vi "Periodic Tasks.vi"(8 "error in":errorcluster) -> ()   [LabVIEW 2013]
doc: "This VI runs in parallel to other tasks. It can contain as many user-defined periodic loops as you need. These can carry out PID or other sorts of timed response."
uses:
  <vilib>/Rock Robotics/WPI/DriverStation/DriverStationLCD/WPI_DriverStationLCDLCDLine.ctl
  <vilib>/Rock Robotics/SystemInterfaces/Utilities/FPGA_UtilitiesLED Source.ctl
  <vilib>/Rock Robotics/SystemInterfaces/Utilities/FPGA_UtilitiesLED State.ctl
  <vilib>/Rock Robotics/WPI/Relay/WPI_RelayValue.ctl
  <vilib>/Rock Robotics/WPI/SafetyOutput/WPI_SafetyOutputConfigMenu.ctl
  <vilib>/Rock Robotics/WPI/DriverStation/WPI_DriverStationRobotMode2.ctl
  <vilib>/Rock Robotics/WPI/Solenoid/WPI_SolenoidValue.ctl
  Begin/Global Refnums.vi
  <vilib>/Rock Robotics/WPI/Solenoid/WPI_SolenoidSetEnum.vi
  Begin/Robot Global Data.vi
  Begin/Global Variables.vi
  <vilib>/Rock Robotics/WPI/Joystick/WPI_JoystickGetSetRefNum.vi
  <vilib>/Rock Robotics/WPI/Compressor/WPI_CompressorGetSetRefNum.vi
panel:
  out "Fire":bool
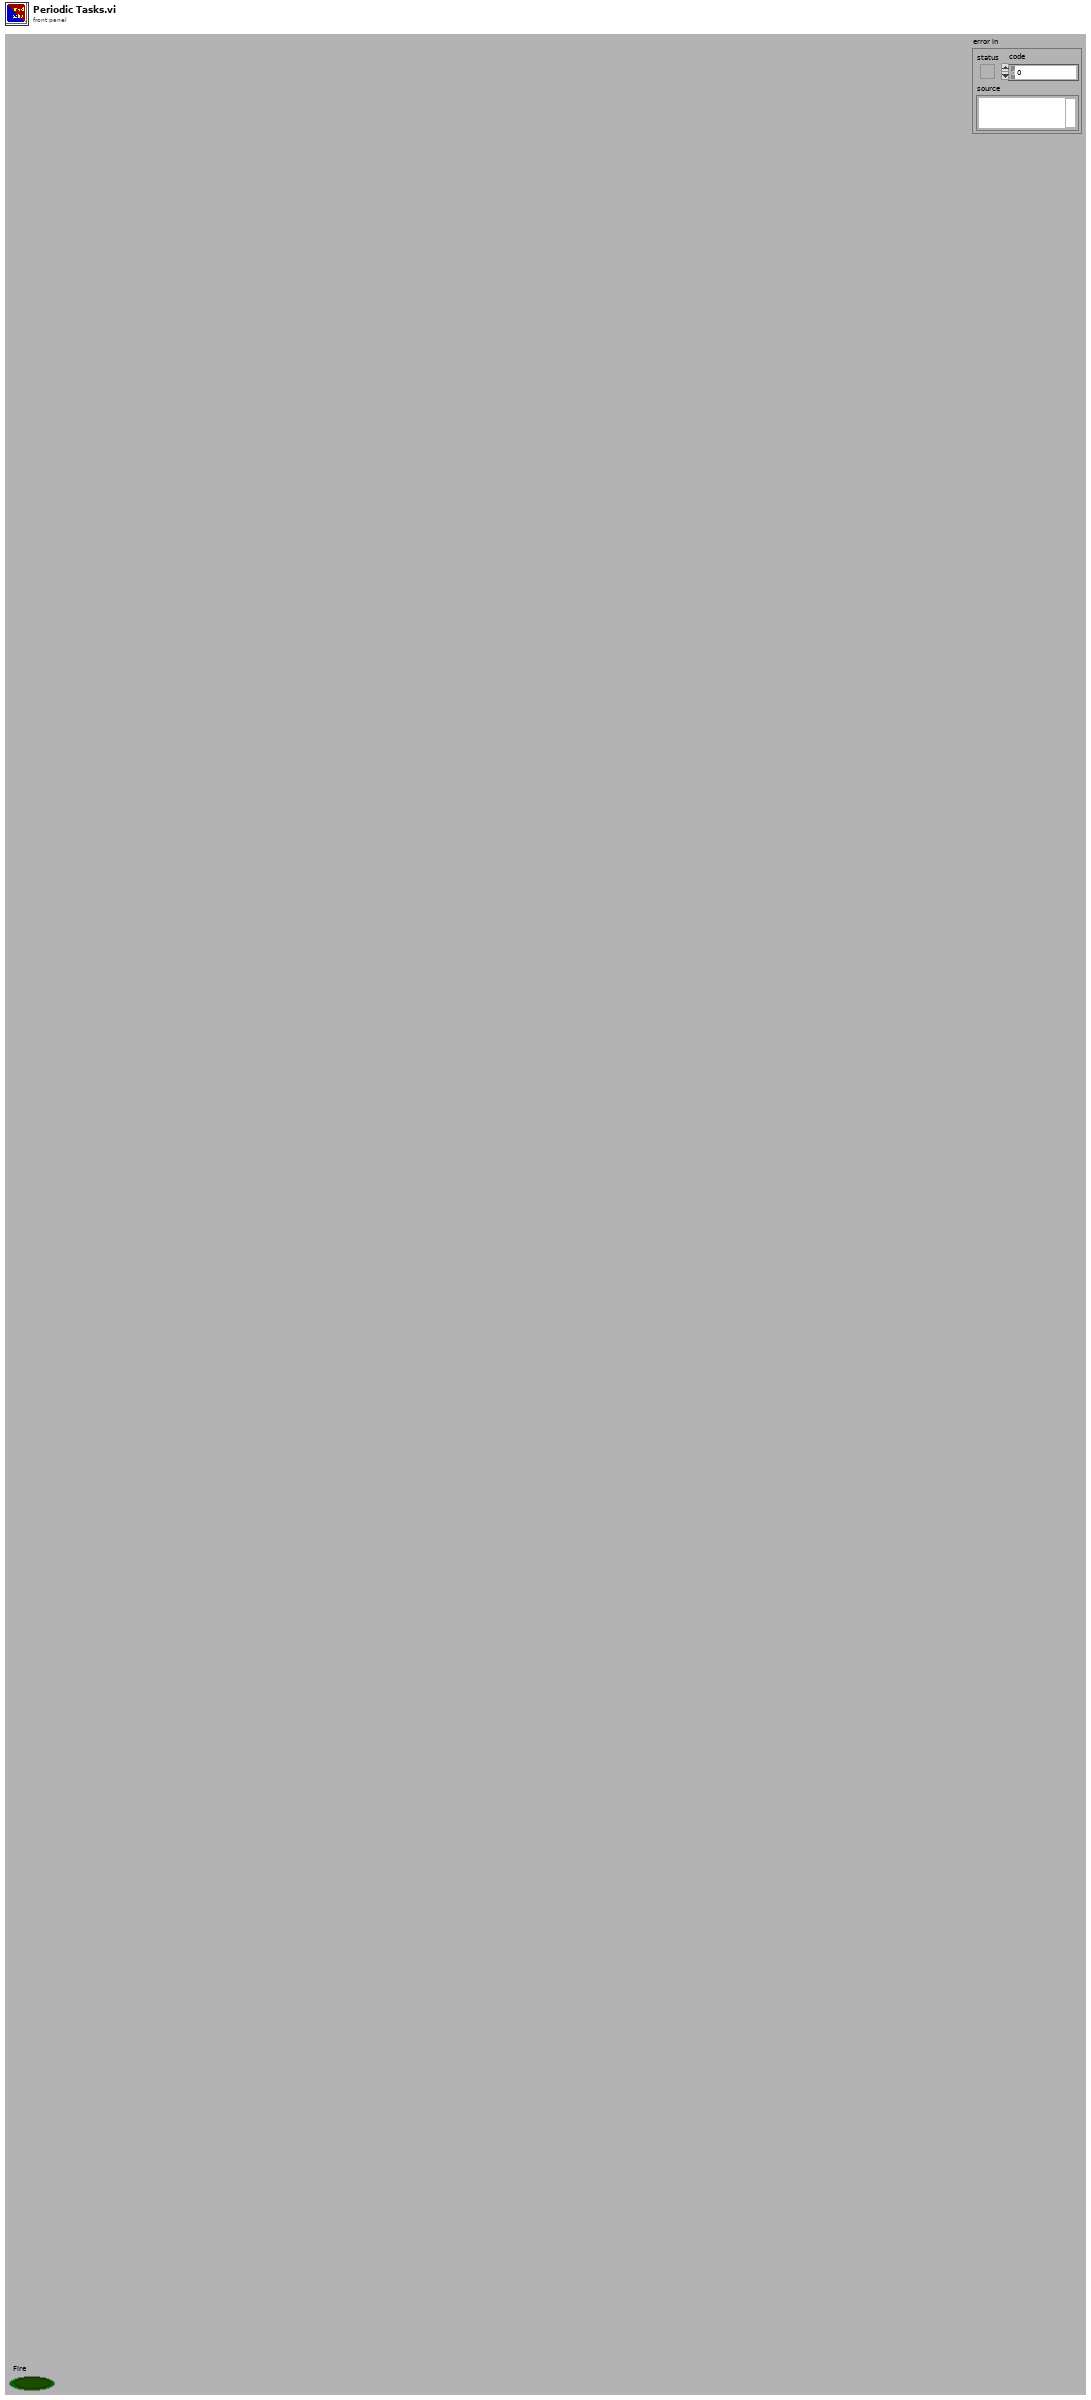
[diagram p1: front panel]
types:
  T1 = typedef "WPI_DriverStationLCDLCDLine.ctl" = enum16{"Main - Line 1", "User - Line 2", "User - Line 3", "User - Line 4", "User - Line 5", "User - Line 6"}
  T2 = typedef "WPI_CompressorDevRef.ctl" = cluster{"DevStatus":errorcluster, "DigitalInputDevRef":T3, "RelayDevRef":T6}
  T3 = typedef "WPI_DigitalInputDevRef.ctl" = cluster{"DevStatus":errorcluster, "DIO Channel":T4, "Digital Module":T5}
  T4 = typedef "FPGA_DIOChannel.ctl" = enum8{"DIO 1", "DIO 2", "DIO 3", "DIO 4", "DIO 5", "DIO 6", "DIO 7", "DIO 8", "DIO 9", "DIO 10", "DIO 11", "DIO 12", "DIO 13", "DIO 14", "Invalid"}
  T5 = typedef "FPGA_TypedefDigitalModule.ctl" = enum16{"Digital Module 1", "Digital Module 2"}
  T6 = typedef "WPI_RelayDevRef.ctl" = cluster{"DevStatus":errorcluster, "Relay Channel":T7, "Digital Module":T5, "Relay Direction":T8}
  T7 = typedef "FPGA_DIORelayChannel.ctl" = enum8{"Relay 1", "Relay 2", "Relay 3", "Relay 4", "Relay 5", "Relay 6", "Relay 7", "Relay 8", "Invalid"}
  T8 = typedef "WPI_RelayDirection.ctl" = enum16{"Both directions", "Forward only", "Reverse only"}
  T9 = typedef "WPI_SolenoidValue.ctl" = enum16{"Off", "On", "Forward", "Reverse"}
  T10 = typedef "WPI_SafetyOutputConfigMenu.ctl" = enum16{"Enable", "Disable"}
  T11 = typedef "WPI_SolenoidDevRef.ctl" = cluster{"DevStatus":errorcluster, "Solenoid Module":T12, "Forward Solenoid Channel":T13, "Reverse Solenoid Channel":T13}
  T12 = typedef "FPGA_TypedefSolenoidModule.ctl" = enum16{"Solenoid Module 1", "Solenoid Module 2"}
  T13 = typedef "WPI_SolenoidChannel.ctl" = enum8{"Solenoid 1", "Solenoid 2", "Solenoid 3", "Solenoid 4", "Solenoid 5", "Solenoid 6", "Solenoid 7", "Solenoid 8", "Invalid"}
  T14 = typedef "WPI_RelayValue.ctl" = enum16{"Off", "On", "Forward", "Reverse"}
  T15 = typedef "WPI_EncoderDevRef.ctl" = cluster{"DevStatus":errorcluster, "EncoderIndex":T16, "CounterIndex":T17, "DistancePerCount":dbl, "Decoding Type":T18}
  T16 = typedef "FPGA_EncoderIdx.ctl" = enum8{"Enc 0", "Enc 1", "Enc 2", "Enc 3", "Invalid"}
  T17 = typedef "FPGA_CounterCtrSystemIndex.ctl" = enum8{"Ctr 0", "Ctr 1", "Ctr 2", "Ctr 3", "Ctr 4", "Ctr 5", "Ctr 6", "Ctr 7", "Invalid"}
  T18 = typedef "WPI_EncoderType.ctl" = enum16{"1x", "2x", "4x"}
  T19 = typedef "WPI_DriverStationRobotMode2.ctl" = enum16{"Autonomous Disabled", "Autonomous Enabled", "Teleop Disabled", "Teleop Enabled", "Timeout", "Finish", "Test Disabled", "Test Enabled"}
  T20 = typedef "WPI_JoystickDevRef.ctl" = cluster{"Device":T21}
  T21 = typedef "WPI_JoystickDeviceEnum.ctl" = enum16{"USB 1", "USB 2", "USB 3", "USB 4", "Kinect 1", "Kinect 2"}
  T22 = typedef "WPI_JoystickButtonState.ctl" = cluster{"Button 1":bool, "Button 2":bool, "Button 3":bool, "Button 4":bool, "Button 5":bool, "Button 6":bool, "Button 7":bool, "Button 8":bool, "Button 9":bool, "Button 10":bool, "Button 11":bool, "Button 12":bool}
  T23 = typedef "WPI_MotorControlDeviceRef.ctl" = cluster{"DeviceStatus":errorcluster, "Type":enum16{"PWM", "CAN"}, "PWM":cluster{"Digital Module":T5, "PWM Channel":T24, "DeadBand":T25}, "CAN":cluster{"Device Number":u8, "Control Mode":T26, "Semaphore":T27, "Max Vout":dbl}, "Invert":bool, "TransformRef":T28, "InvTransformRef":T28}
  T24 = typedef "FPGA_DIOPWMChannel.ctl" = enum8{"PWM 1", "PWM 2", "PWM 3", "PWM 4", "PWM 5", "PWM 6", "PWM 7", "PWM 8", "PWM 9", "PWM 10", "Invalid"}
  T25 = typedef "WPI_PWMDeadband.ctl" = cluster{"Name":string, "maxPositivePwm":i32, "minPositivePwm":i32, "centerPwm":i32, "maxNegativePwm":i32, "minNegativePwm":i32, "angularRange":u16}
  T26 = typedef "WPI_CANJaguar_ControlMode.ctl" = enum8{"Percent VBus", "Current", "Speed", "Position", "Voltage"}
  T27 = typedef "Semaphore RefNum" = refnum<k1>
  T28 = typedef "WPI_PWMTransform_ConPane.ctl" = refnum<vi>
  T29 = typedef "FPGA_UtilitiesLED State.ctl" = enum16{"Off", "On", "Toggle"}
  T30 = typedef "FPGA_UtilitiesLED Source.ctl" = enum16{"User LED", "FPGA LED"}
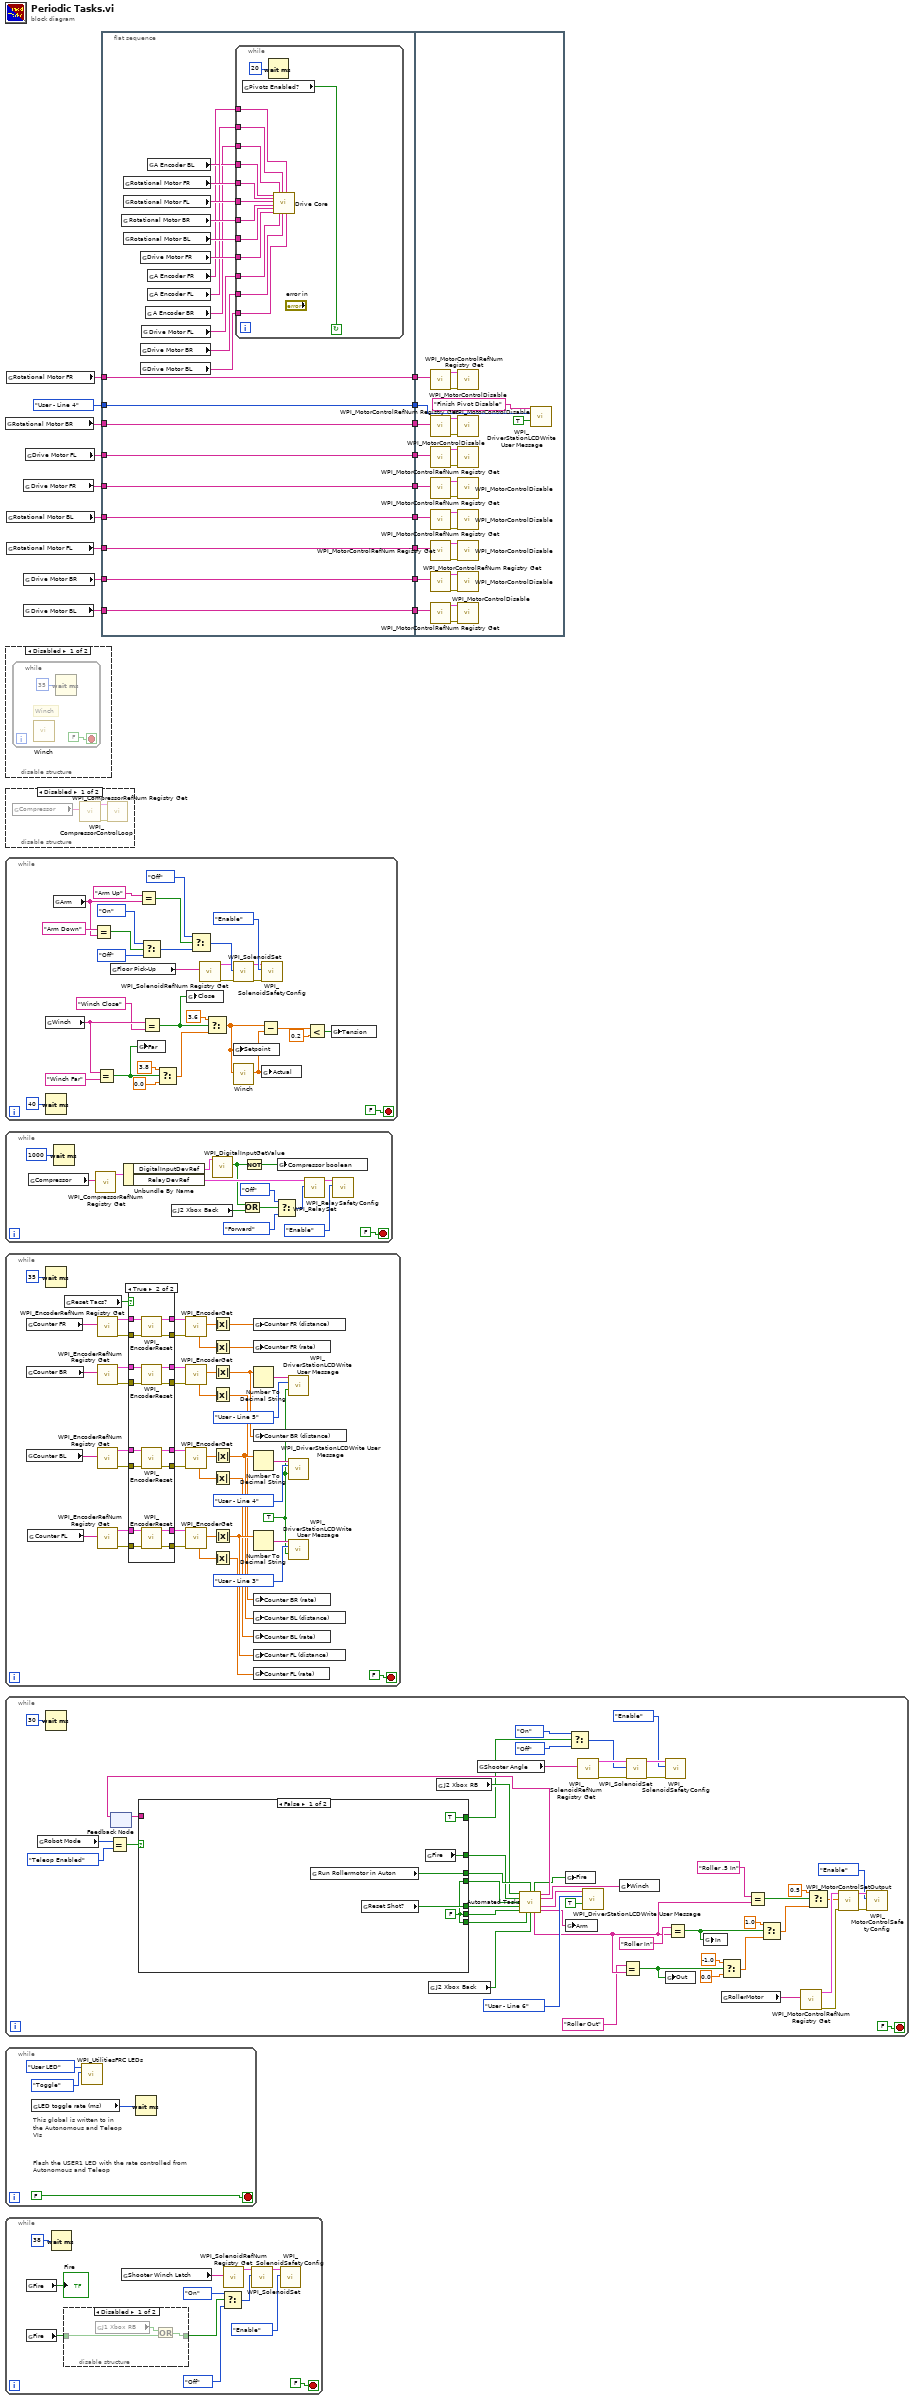
[diagram p0: block diagram]
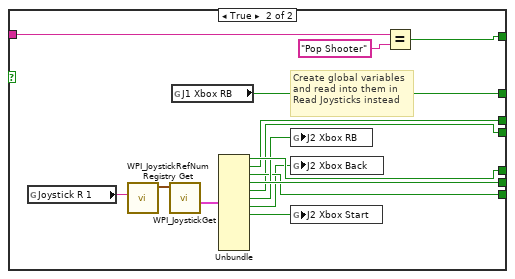
[diagram p4: hidden frame]
diagram:
  n1 = global read "Global Refnums.vi" "Rotational Motor BR"() -> (w16:string)
  n2 = disable-structure shown="Disabled" {
    frame Disabled {
      n3 = while {
        stop <- FALSE stop-if-true
        # "Winch"
        n4 = call "Winch.vi"() -> ()  [unwired: 11 in, 1 out]
        n5 = Wait (ms)(milliseconds to wait=u32 35) -> ()  [unwired: 1 out]
      }
    }
    frame Enabled {
    }
  }
  n6 = disable-structure shown="Disabled" {
    frame Disabled {
      n7 = global read "Global Refnums.vi" "Compressor"() -> (w23:string)
      n8 = call <vilib>:"WPI_CompressorRefNum Registry Get.vi"("refnum name"=w23) -> ("error out"=w22:errorcluster, "CompressorDevRef"=w21:T2)  [unwired: 9 in]
      n9 = call <vilib>:"WPI_CompressorControlLoop.vi"("error in (no error)"=w22, "CompressorDevRef"=w21) -> ()  [unwired: 10 in]
    }
    frame Enabled {
    }
  }
  n10 = while {
    stop <- FALSE stop-if-true
    n11 = global read "Global Refnums.vi" "Winch"() -> (w55:string)
    n12 = Wait (ms)(milliseconds to wait=u32 40) -> ()  [unwired: 1 out]
    n13 = global read "Global Refnums.vi" "Arm"() -> (w29:string)
    n14 = Equal?(x="Arm Down", y=w29) -> (x = y?=w33:bool)
    n15 = Equal?(x=w55, y="Winch Far") -> (x = y?=w26:bool)
    n16 = global read "Global Refnums.vi" "Floor Pick-Up"() -> (w44:string)
    n17 = global write "Global Refnums.vi" "Far"(w26) -> ()
    n18 = Equal?(x="Arm Up", y=w29) -> (x = y?=w46:bool)
    n19 = Select(t=WPI_SolenoidValue."On" ("Value"), s=w33, f=WPI_SolenoidValue."Off" ("Value")) -> (s? t:f=w32:T9)
    n20 = Equal?(x=w55, y="Winch Close") -> (x = y?=w25:bool)
    n21 = Select(t=3.8, s=w26, f=0.0) -> (s? t:f=w52:dbl)
    n22 = global write "Global Refnums.vi" "Close"(w25) -> ()
    n23 = Select(t=WPI_SolenoidValue."Off" ("Value"), s=w46, f=w32) -> (s? t:f=w48:T9)
    n24 = call <vilib>:"WPI_SolenoidRefNum Registry Get.vi"("refnum name"=w44) -> ("error out"=w39:errorcluster, "SolenoidDevRef"=w40:T11)  [unwired: 9 in]
    n25 = Select(t=3.6, s=w25, f=w52) -> (s? t:f=w24:dbl)
    n26 = call-poly <vilib>:"WPI_SolenoidSet.vi"("error in (no error)"=w39, "Value"=w48, "SolenoidDevRef"=w40) -> ("error out"=w42:errorcluster, "SolenoidDevRef"=w41:T11)  [unwired: 7 in]
    n27 = global write "Global Refnums.vi" "Setpoint"(w24) -> ()
    n28 = call "Winch.vi"("setpoint"=w24) -> ("Actual"=w27:dbl)  [unwired: 10 in]
    n29 = Subtract(x=w24, y=w27) -> (x-y=w36:dbl)
    n30 = call <vilib>:"WPI_SolenoidSafetyConfig.vi"("error in (no error)"=w42, "mode"=WPI_SafetyOutputConfigMenu."Enable", "SolenoidDevRef"=w41) -> ()  [unwired: 7 in, 2 out]
    n31 = global write "Global Refnums.vi" "Actual"(w27) -> ()
    n32 = Less?(x=w36, y=0.2) -> (x < y?=w28:bool)
    n33 = global write "Global Refnums.vi" "Tension"(w28) -> ()
  }
  n34 = while {
    stop <- FALSE stop-if-true
    n35 = global read "Global Refnums.vi" "Compressor"() -> (w68:string)
    n36 = Wait (ms)(milliseconds to wait=1000) -> ()  [unwired: 1 out]
    n37 = call <vilib>:"WPI_CompressorRefNum Registry Get.vi"("refnum name"=w68) -> ("CompressorDevRef"=w67:T2)  [unwired: 9 in, 1 out]
    n38 = Unbundle By Name(w67) -> ("DigitalInputDevRef"=w60:T3, "RelayDevRef"=w66:T6)
    n39 = global read "Global Variables.vi" "J2 Xbox Back"() -> (w58:bool)
    n40 = call <vilib>:"WPI_DigitalInputGetValue.vi"("DigitalInputDevRef"=w60) -> ("Value"=w57:bool)  [unwired: 8 in, 2 out]
    n41 = Or(x=w57, y=w58) -> (x .or. y?=w59:bool)
    n42 = Not(x=w57) -> (.not. x?=w56:bool)
    n43 = Select(t=WPI_RelayValue."Off" ("RelayValue"), s=w59, f=WPI_RelayValue."Forward" ("RelayValue")) -> (s? t:f=w63:T14)
    n44 = global write "Global Refnums.vi" "Compressor boolean"(w56) -> ()
    n45 = call <vilib>:"WPI_RelaySet.vi"("RelayValue"=w63, "RelayDevRef"=w66) -> ("RelayDevRef"=w65:T6)  [unwired: 8 in, 1 out]
    n46 = call <vilib>:"WPI_RelaySafetyConfig.vi"("mode"=WPI_SafetyOutputConfigMenu."Enable", "RelayDevRef"=w65) -> ()  [unwired: 8 in, 2 out]
  }
  n47 = while {
    stop <- FALSE stop-if-true
    w72 = TRUE ("clear line before write (T)")
    n48 = global read "Global Refnums.vi" "Counter FR"() -> (w83:string)
    n49 = global read "Global Refnums.vi" "Counter BR"() -> (w81:string)
    n50 = global read "Global Refnums.vi" "Counter BL"() -> (w84:string)
    n51 = global read "Global Refnums.vi" "Counter FL"() -> (w82:string)
    n52 = Wait (ms)(milliseconds to wait=u32 35) -> ()  [unwired: 1 out]
    n53 = global read "Global Variables.vi" "Reset Tacs?"() -> (w71:bool)
    n54 = call <vilib>:"WPI_EncoderRefNum Registry Get.vi"("refnum name"=w83) -> ("error out"=w99:errorcluster, "EncoderDevRef"=w102:T15)  [unwired: 9 in]
    n55 = call <vilib>:"WPI_EncoderRefNum Registry Get.vi"("refnum name"=w81) -> ("error out"=w107:errorcluster, "EncoderDevRef"=w108:T15)  [unwired: 9 in]
    n56 = call <vilib>:"WPI_EncoderRefNum Registry Get.vi"("refnum name"=w84) -> ("error out"=w109:errorcluster, "EncoderDevRef"=w110:T15)  [unwired: 9 in]
    n57 = call <vilib>:"WPI_EncoderRefNum Registry Get.vi"("refnum name"=w82) -> ("error out"=w104:errorcluster, "EncoderDevRef"=w105:T15)  [unwired: 9 in]
    n58 = case shown="True" w71 {
      tunnel: w108 -> [w121 w140]
      tunnel: [w121 w139] -> w113
      tunnel: [w123 w138] -> w114
      tunnel: w107 -> [w123 w137]
      tunnel: [w122 w136] -> w112
      tunnel: [w124 w135] -> w111
      tunnel: w110 -> [w122 w134]
      tunnel: w109 -> [w124 w133]
      tunnel: [w120 w125] -> w106
      tunnel: w105 -> [w120 w132]
      tunnel: w104 -> [w119 w131]
      tunnel: [w119 w126] -> w103
      tunnel: w102 -> [w118 w130]
      tunnel: [w118 w127] -> w101
      tunnel: [w117 w128] -> w100
      tunnel: w99 -> [w117 w129]
      frame False {
      }
      frame True {
        n59 = call <vilib>:"WPI_EncoderReset.vi"("error in (no error)"=w129, "EncoderDevRef"=w130) -> ("error out"=w128:errorcluster, "EncoderDevRef"=w127:T15)  [unwired: 8 in]
        n60 = call <vilib>:"WPI_EncoderReset.vi"("error in (no error)"=w137, "EncoderDevRef"=w140) -> ("error out"=w138:errorcluster, "EncoderDevRef"=w139:T15)  [unwired: 8 in]
        n61 = call <vilib>:"WPI_EncoderReset.vi"("error in (no error)"=w133, "EncoderDevRef"=w134) -> ("error out"=w135:errorcluster, "EncoderDevRef"=w136:T15)  [unwired: 8 in]
        n62 = call <vilib>:"WPI_EncoderReset.vi"("error in (no error)"=w131, "EncoderDevRef"=w132) -> ("error out"=w126:errorcluster, "EncoderDevRef"=w125:T15)  [unwired: 8 in]
      }
    }
    n63 = call <vilib>:"WPI_EncoderGet.vi"("error in (no error)"=w100, "EncoderDevRef"=w101) -> ("Distance"=w96:dbl, "Rate"=w92:dbl)  [unwired: 4 in, 4 out]
    n64 = call <vilib>:"WPI_EncoderGet.vi"("error in (no error)"=w114, "EncoderDevRef"=w113) -> ("Distance"=w95:dbl, "Rate"=w91:dbl)  [unwired: 4 in, 4 out]
    n65 = call <vilib>:"WPI_EncoderGet.vi"("error in (no error)"=w111, "EncoderDevRef"=w112) -> ("Distance"=w97:dbl, "Rate"=w93:dbl)  [unwired: 4 in, 4 out]
    n66 = call <vilib>:"WPI_EncoderGet.vi"("error in (no error)"=w103, "EncoderDevRef"=w106) -> ("Distance"=w98:dbl, "Rate"=w94:dbl)  [unwired: 4 in, 4 out]
    n67 = Absolute Value(x=w96) -> (abs(x)=w80:dbl)
    n68 = Absolute Value(x=w92) -> (abs(x)=w79:dbl)
    n69 = Absolute Value(x=w91) -> (abs(x)=w73:dbl)
    n70 = Absolute Value(x=w93) -> (abs(x)=w75:dbl)
    n71 = Absolute Value(x=w94) -> (abs(x)=w77:dbl)
    n72 = Absolute Value(x=w95) -> (abs(x)=w74:dbl)
    n73 = Absolute Value(x=w97) -> (abs(x)=w76:dbl)
    n74 = Absolute Value(x=w98) -> (abs(x)=w78:dbl)
    n75 = global write "Global Refnums.vi" "Counter FR (distance)"(w80) -> ()
    n76 = global write "Global Refnums.vi" "Counter FR (rate)"(w79) -> ()
    n77 = Number To Decimal String(number=w74) -> (decimal integer string=w90:string)  [unwired: 1 in]
    n78 = global write "Global Refnums.vi" "Counter BR (distance)"(w74) -> ()
    n79 = Number To Decimal String(number=w76) -> (decimal integer string=w88:string)  [unwired: 1 in]
    n80 = Number To Decimal String(number=w78) -> (decimal integer string=w89:string)  [unwired: 1 in]
    n81 = global write "Global Refnums.vi" "Counter BR (rate)"(w73) -> ()
    n82 = global write "Global Refnums.vi" "Counter BL (distance)"(w76) -> ()
    n83 = global write "Global Refnums.vi" "Counter BL (rate)"(w75) -> ()
    n84 = global write "Global Refnums.vi" "Counter FL (distance)"(w78) -> ()
    n85 = global write "Global Refnums.vi" "Counter FL (rate)"(w77) -> ()
    n86 = call <vilib>:"WPI_DriverStationLCDWrite User Message.vi"("line text"=w90, "line"=WPI_DriverStationLCDLCDLine."User - Line 5", "clear line before write (T)"=w72) -> ()  [unwired: 12 in, 1 out]
    n87 = call <vilib>:"WPI_DriverStationLCDWrite User Message.vi"("line text"=w88, "line"=WPI_DriverStationLCDLCDLine."User - Line 4", "clear line before write (T)"=w72) -> ()  [unwired: 12 in, 1 out]
    n88 = call <vilib>:"WPI_DriverStationLCDWrite User Message.vi"("line text"=w89, "line"=WPI_DriverStationLCDLCDLine."User - Line 3", "clear line before write (T)"=w72) -> ()  [unwired: 12 in, 1 out]
  }
  n89 = while {
    stop <- FALSE stop-if-true
    n90 = global read "Robot Global Data.vi" "Robot Mode"() -> (w162:T19)
    n91 = Wait (ms)(milliseconds to wait=u32 30) -> ()  [unwired: 1 out]
    n92 = Equal?(x=w162, y=WPI_DriverStationRobotMode2."Teleop Enabled") -> (x = y?=w163:bool)
    n93 = feedback #1() -> (w158:string)  [unwired: 1 in]
    n94 = case shown="False" w163 {
      tunnel: [w193 w208] -> w146
      tunnel: [w195 w207] -> w174
      tunnel: [w192 w206] -> w173
      tunnel: [w196 w205] -> w172
      tunnel: w158 -> [_ w203]
      tunnel: [TRUE w202] -> w157
      tunnel: [w192 w200] -> w155
      tunnel: [w192 w199] -> w147
      frame False {
        w192 = FALSE ("J1 Xbox RB")
        n95 = global read "Global Refnums.vi" "Run Rollermotor in Auton"() -> (w195:bool)
        n96 = global read "Global Refnums.vi" "Reset Shot?"() -> (w193:bool)
        n97 = global read "Global Refnums.vi" "Fire"() -> (w196:bool)
      }
      frame True {
        # "Create global variables\nand read into them in \nRead Joysticks instead"
        n98 = global read "Global Refnums.vi" "Joystick R 1"() -> (w209:string)
        n99 = call <vilib>:"WPI_JoystickRefNum Registry Get.vi"("refnum name"=w209) -> ("JoystickDevRef"=w211:T20)  [unwired: 9 in, 1 out]
        n100 = call <vilib>:"WPI_JoystickGet.vi"("JoystickDevRef"=w211) -> ("Buttons"=w210:T22)  [unwired: 4 in, 2 out]
        n101 = global read "Global Variables.vi" "J1 Xbox RB"() -> (w205:bool)
        n102 = Unbundle(w210) -> ("Button 1"=w208:bool, "Button 2"=w207:bool, "Button 3"=w200:bool, "Button 4"=w206:bool, "Button 5"=w199:bool, "Button 6"=w201:bool, "Button 7"=w198:bool, "Button 8"=w197:bool)  [unwired: 4 out]
        n103 = global write "Global Variables.vi" "J2 Xbox RB"(w201) -> ()
        n104 = global write "Global Variables.vi" "J2 Xbox Back"(w198) -> ()
        n105 = global write "Global Variables.vi" "J2 Xbox Start"(w197) -> ()
        n106 = Equal?(x=w203, y="Pop Shooter") -> (x = y?=w202:bool)
      }
    }
    n107 = global read "Global Variables.vi" "J2 Xbox Back"() -> (w143:bool)
    n108 = global read "Global Variables.vi" "J2 Xbox RB"() -> (w160:bool)
    n109 = global read "Global Refnums.vi" "Shooter Angle"() -> (w170:string)
    n110 = call "Automated Tasks.vi"("RB"=w160, "B"=w174, "Fire"=w172, "LB"=w147, "A"=w146, "Y"=w173, "X"=w155, "Back"=w143) -> ("Fire"=w156:bool, "Shooter"=w159:string, "Winch"=w145:string, "Case"=w168:string, "Roller"=w152:string, "Arm"=w165:string)  [unwired: 2 in]
    n111 = feedback-in #1(w159) -> ()
    n112 = global write "Global Refnums.vi" "Fire"(w156) -> ()
    n113 = global write "Global Refnums.vi" "Arm"(w165) -> ()
    n114 = Select(t=WPI_SolenoidValue."On" ("Value"), s=w157, f=WPI_SolenoidValue."Off" ("Value")) -> (s? t:f=w175:T9)
    n115 = call <vilib>:"WPI_SolenoidRefNum Registry Get.vi"("refnum name"=w170) -> ("error out"=w182:errorcluster, "SolenoidDevRef"=w181:T11)  [unwired: 9 in]
    n116 = call <vilib>:"WPI_DriverStationLCDWrite User Message.vi"("line text"=w168, "line"=WPI_DriverStationLCDLCDLine."User - Line 6", "clear line before write (T)"=TRUE) -> ()  [unwired: 12 in, 1 out]
    n117 = global write "Global Refnums.vi" "Winch"(w145) -> ()
    n118 = Equal?(x="Roller Out", y=w152) -> (x = y?=w141:bool)
    n119 = call-poly <vilib>:"WPI_SolenoidSet.vi"("error in (no error)"=w182, "Value"=w175, "SolenoidDevRef"=w181) -> ("error out"=w179:errorcluster, "SolenoidDevRef"=w180:T11)  [unwired: 7 in]
    n120 = call <vilib>:"WPI_SolenoidSafetyConfig.vi"("error in (no error)"=w179, "mode"=WPI_SafetyOutputConfigMenu."Enable", "SolenoidDevRef"=w180) -> ()  [unwired: 7 in, 2 out]
    n121 = global write "Global Refnums.vi" "Out"(w141) -> ()
    n122 = Equal?(x="Roller In", y=w152) -> (x = y?=w142:bool)
    n123 = global write "Global Refnums.vi" "In"(w142) -> ()
    n124 = Select(t=-1.0, s=w141, f=0.0) -> (s? t:f=w183:dbl)
    n125 = global read "Global Refnums.vi" "RollerMotor"() -> (w171:string)
    n126 = Equal?(x="Roller .5 In", y=w152) -> (x = y?=w151:bool)
    n127 = Select(t=1.0, s=w142, f=w183) -> (s? t:f=w150:dbl)
    n128 = call <vilib>:"WPI_MotorControlRefNum Registry Get.vi"("refnum name"=w171) -> ("error out"=w189:errorcluster, "MotorControlDevRef"=w191:T23)  [unwired: 9 in]
    n129 = Select(t=0.5, s=w151, f=w150) -> (s? t:f=w154:dbl)
    n130 = call <vilib>:"WPI_MotorControlSetOutput.vi"("error in (no error)"=w189, "Output"=w154, "MotorControlDevRef"=w191) -> ("error out"=w188:errorcluster, "MotorControlDevRef"=w190:T23)  [unwired: 6 in, 1 out]
    n131 = call <vilib>:"WPI_MotorControlSafetyConfig.vi"("error in (no error)"=w188, "mode"=WPI_SafetyOutputConfigMenu."Enable", "MotorControlDevRef"=w190) -> ()  [unwired: 7 in, 2 out]
  }
  n132 = while {
    stop <- FALSE stop-if-true
    # "This global is written to in the Autonomous and Teleop VIs"
    # "Flash the USER1 LED with the rate controlled from Autonomous and Teleop"
    n133 = global read "Robot Global Data.vi" "LED toggle rate (ms)"() -> (w212:u32)
    n134 = call <vilib>:"WPI_UtilitiesFRC LEDs.vi"("State"=FPGA_UtilitiesLED_State."Toggle", "LED Type"=FPGA_UtilitiesLED_Source."User LED") -> ()  [unwired: 1 in, 9 out]
    n135 = Wait (ms)(milliseconds to wait=w212) -> ()  [unwired: 1 out]
  }
  n136 = while {
    stop <- FALSE stop-if-true
    n137 = global read "Global Refnums.vi" "Fire"() -> (→"Fire":bool)
    n138 = global read "Global Refnums.vi" "Fire"() -> (w217:bool)
    n139 = Wait (ms)(milliseconds to wait=u32 38) -> ()  [unwired: 1 out]
    n140 = disable-structure shown="Disabled" {
      disable-tunnel: w217 -> [w230 w231]
      disable-tunnel: [w228 w231] -> w216
      frame Disabled {
        n141 = global read "Global Variables.vi" "J1 Xbox RB"() -> (w229:bool)
        n142 = Or(x=w229, y=w230) -> (x .or. y?=w228:bool)
      }
      frame Enabled {
      }
    }
    n143 = global read "Global Refnums.vi" "Shooter Winch Latch"() -> (w223:string)
    n144 = Select(t=WPI_SolenoidValue."On", s=w216, f=WPI_SolenoidValue."Off" ("Value")) -> (s? t:f=w218:T9)
    n145 = call <vilib>:"WPI_SolenoidRefNum Registry Get.vi"("refnum name"=w223) -> ("SolenoidDevRef"=w224:T11)  [unwired: 9 in, 1 out]
    n146 = call-poly <vilib>:"WPI_SolenoidSet.vi"("Value"=w218, "SolenoidDevRef"=w224) -> ("SolenoidDevRef"=w225:T11)  [unwired: 8 in, 1 out]
    n147 = call <vilib>:"WPI_SolenoidSafetyConfig.vi"("mode"=WPI_SafetyOutputConfigMenu."Enable", "SolenoidDevRef"=w225) -> ()  [unwired: 8 in, 2 out]
  }
  n148 = global read "Global Refnums.vi" "Rotational Motor FR"() -> (w18:string)
  n149 = global read "Global Refnums.vi" "Rotational Motor BL"() -> (w15:string)
  n150 = global read "Global Refnums.vi" "Rotational Motor FL"() -> (w17:string)
  n151 = global read "Global Refnums.vi" "Drive Motor FR"() -> (w14:string)
  n152 = global read "Global Refnums.vi" "Drive Motor BR"() -> (w12:string)
  n153 = global read "Global Refnums.vi" "Drive Motor BL"() -> (w11:string)
  n154 = global read "Global Refnums.vi" "Drive Motor FL"() -> (w13:string)
  n155 = flat-sequence {
    tunnel: WPI_DriverStationLCDLCDLine."User - Line 4" ("line") -> [w244]
    tunnel: w13 -> [w245]
    tunnel: w11 -> [w246]
    tunnel: w12 -> [w247]
    tunnel: w14 -> [w248]
    tunnel: w15 -> [w249]
    tunnel: w16 -> [w250]
    tunnel: w17 -> [w251]
    tunnel: w18 -> [w252]
    tunnel: [w252] -> w9
    tunnel: [w251] -> w8
    tunnel: [w250] -> w7
    tunnel: [w249] -> w6
    tunnel: [w248] -> w5
    tunnel: [w247] -> w4
    tunnel: [w246] -> w3
    tunnel: [w245] -> w2
    tunnel: [w244] -> w1
    tunnel: w9 -> [w293]
    tunnel: w8 -> [w286]
    tunnel: w7 -> [w285]
    tunnel: w6 -> [w282]
    tunnel: w5 -> [w273]
    tunnel: w4 -> [w272]
    tunnel: w3 -> [w271]
    tunnel: w2 -> [w270]
    tunnel: w1 -> [w269]
    frame #0 {
      n156 = global read "Global Refnums.vi" "Rotational Motor BR"() -> (w238:string)
      n157 = global read "Global Refnums.vi" "Rotational Motor FR"() -> (w236:string)
      n158 = global read "Global Refnums.vi" "Rotational Motor FL"() -> (w237:string)
      n159 = global read "Global Refnums.vi" "Rotational Motor BL"() -> (w239:string)
      n160 = global read "Global Refnums.vi" "Drive Motor FR"() -> (w240:string)
      n161 = global read "Global Refnums.vi" "Drive Motor BR"() -> (w242:string)
      n162 = global read "Global Refnums.vi" "Drive Motor BL"() -> (w243:string)
      n163 = global read "Global Refnums.vi" "Drive Motor FL"() -> (w241:string)
      n164 = global read "Global Refnums.vi" "A Encoder BR"() -> (w233:string)
      n165 = global read "Global Refnums.vi" "A Encoder BL"() -> (w234:string)
      n166 = global read "Global Refnums.vi" "A Encoder FR"() -> (w232:string)
      n167 = global read "Global Refnums.vi" "A Encoder FL"() -> (w235:string)
      n168 = while {
        tunnel: w232 -> [w266]
        tunnel: w233 -> [w264]
        tunnel: w234 -> [w263]
        tunnel: w235 -> [w265]
        tunnel: w240 -> [w258]
        tunnel: w242 -> [w256]
        tunnel: w243 -> [w255]
        tunnel: w241 -> [w257]
        tunnel: w236 -> [w262]
        tunnel: w238 -> [w260]
        tunnel: w239 -> [w259]
        tunnel: w237 -> [w261]
        stop <- w253 continue-if-true
        n169 = global read "Global Variables.vi" "Pivots Enabled?"() -> (w253:bool)
        n170 = Wait (ms)(milliseconds to wait=u32 20) -> ()  [unwired: 1 out]
        n171 = call "Drive Core.vi"("A Encoder BL"=w263, "Rotational Motor FR"=w262, "Rotational Motor FL"=w261, "Rotational Motor BR"=w260, "Rotational Motor BL"=w259, "Drive Motor FR"=w258, "A Encoder BR"=w264, "Drive Motor FL"=w257, "A Encoder FL"=w265, "Drive Motor BR"=w256, "A Encoder FR"=w266, "Drive Motor BL"=w255) -> ()  [unwired: 8 in]
      }
    }
    frame #1 {
      n172 = call <vilib>:"WPI_MotorControlRefNum Registry Get.vi"("refnum name"=w293) -> ("error out"=w291:errorcluster, "MotorControlDevRef"=w292:T23)  [unwired: 9 in]
      n173 = call <vilib>:"WPI_MotorControlRefNum Registry Get.vi"("refnum name"=w285) -> ("error out"=w287:errorcluster, "MotorControlDevRef"=w288:T23)  [unwired: 9 in]
      n174 = call <vilib>:"WPI_MotorControlRefNum Registry Get.vi"("refnum name"=w270) -> ("error out"=w277:errorcluster, "MotorControlDevRef"=w276:T23)  [unwired: 9 in]
      n175 = call <vilib>:"WPI_MotorControlRefNum Registry Get.vi"("refnum name"=w273) -> ("error out"=w275:errorcluster, "MotorControlDevRef"=w274:T23)  [unwired: 9 in]
      n176 = call <vilib>:"WPI_MotorControlRefNum Registry Get.vi"("refnum name"=w282) -> ("error out"=w283:errorcluster, "MotorControlDevRef"=w284:T23)  [unwired: 9 in]
      n177 = call <vilib>:"WPI_MotorControlRefNum Registry Get.vi"("refnum name"=w286) -> ("error out"=w289:errorcluster, "MotorControlDevRef"=w290:T23)  [unwired: 9 in]
      n178 = call <vilib>:"WPI_MotorControlRefNum Registry Get.vi"("refnum name"=w272) -> ("error out"=w279:errorcluster, "MotorControlDevRef"=w278:T23)  [unwired: 9 in]
      n179 = call <vilib>:"WPI_MotorControlRefNum Registry Get.vi"("refnum name"=w271) -> ("error out"=w281:errorcluster, "MotorControlDevRef"=w280:T23)  [unwired: 9 in]
      n180 = call <vilib>:"WPI_MotorControlDisable.vi"("error in (no error)"=w291, "MotorControlDevRef"=w292) -> ()  [unwired: 8 in, 2 out]
      n181 = call <vilib>:"WPI_MotorControlDisable.vi"("error in (no error)"=w287, "MotorControlDevRef"=w288) -> ()  [unwired: 8 in, 2 out]
      n182 = call <vilib>:"WPI_MotorControlDisable.vi"("error in (no error)"=w277, "MotorControlDevRef"=w276) -> ()  [unwired: 8 in, 2 out]
      n183 = call <vilib>:"WPI_MotorControlDisable.vi"("error in (no error)"=w275, "MotorControlDevRef"=w274) -> ()  [unwired: 8 in, 2 out]
      n184 = call <vilib>:"WPI_MotorControlDisable.vi"("error in (no error)"=w283, "MotorControlDevRef"=w284) -> ()  [unwired: 8 in, 2 out]
      n185 = call <vilib>:"WPI_MotorControlDisable.vi"("error in (no error)"=w289, "MotorControlDevRef"=w290) -> ()  [unwired: 8 in, 2 out]
      n186 = call <vilib>:"WPI_MotorControlDisable.vi"("error in (no error)"=w279, "MotorControlDevRef"=w278) -> ()  [unwired: 8 in, 2 out]
      n187 = call <vilib>:"WPI_MotorControlDisable.vi"("error in (no error)"=w281, "MotorControlDevRef"=w280) -> ()  [unwired: 8 in, 2 out]
      n188 = call <vilib>:"WPI_DriverStationLCDWrite User Message.vi"("line text"="Finish Pivot Disable", "line"=w269, "clear line before write (T)"=TRUE) -> ()  [unwired: 12 in, 1 out]
    }
  }
